vi "Debug Exercise (Main) SOLVED.vi"() -> ()   [LabVIEW 2015]
doc: "This VI is an exercise in the LabVIEW Basics I course.\n\nThis exercise is used to demonstrate the use of different debugging tools. First, fix the broken run arrow and then use the different debugging tools to see how they work."
panel:
  out "Final Result":dbl format="%.2f"
  out "Random Number":dbl format="%.2f"
  out "Multiply Result":dbl format="%.2f"
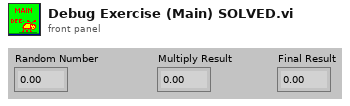
[diagram p1: front panel]
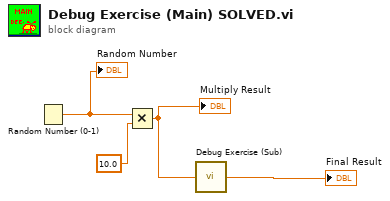
[diagram p0: block diagram]
diagram:
  n1 = Random Number (0-1)() -> (number: 0 to 1=w4:dbl)
  "Random Number" <- w4
  n2 = Multiply(x=w4, y=10.0) -> (x*y=w1:dbl)
  "Multiply Result" <- w1
  n3 = call "Debug Exercise (Sub).vi"("Number"=w1) -> ("Final Result"=→"Final Result":dbl)
